vi "testCreate.vi"(8 "error in (no error)":errorcluster, 11 "TestCase in":refnum<class "StringList_Delegations.lvclass">) -> (0 "error out":errorcluster, 3 "TestCase out":refnum<class "StringList_Delegations.lvclass">)   [LabVIEW 2013, in "StringList_Delegations.lvclass"]
uses:
  StringList_Delegations.lvclass
  StringList_Delegations.lvclass/StringList_Delegations.ctl
  <vilib>/addons/_JKI Toolkits/VI Tester/TestCase.llb/TestCase.lvclass
  UnitTestComparisons/UnitTestComparisons.lvlib
  Test Doubles/ListImp_RefSpy/ListImp_RefSpy.lvclass
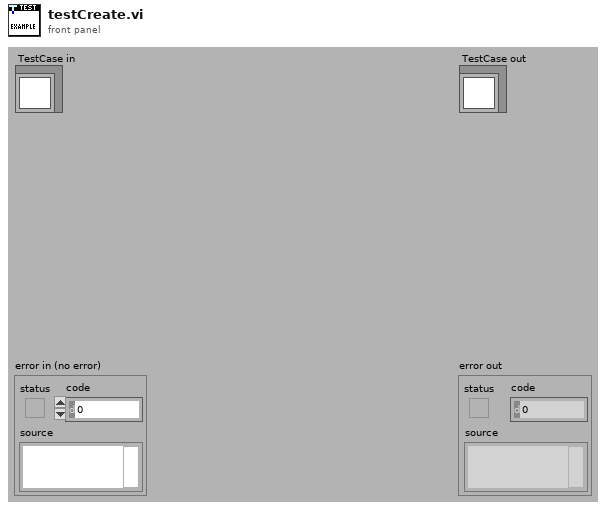
[diagram p1: front panel]
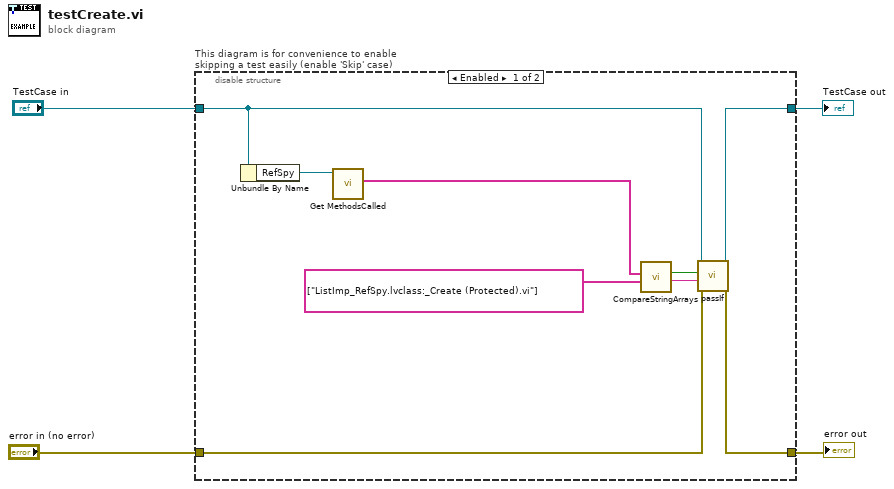
[diagram p0: block diagram]
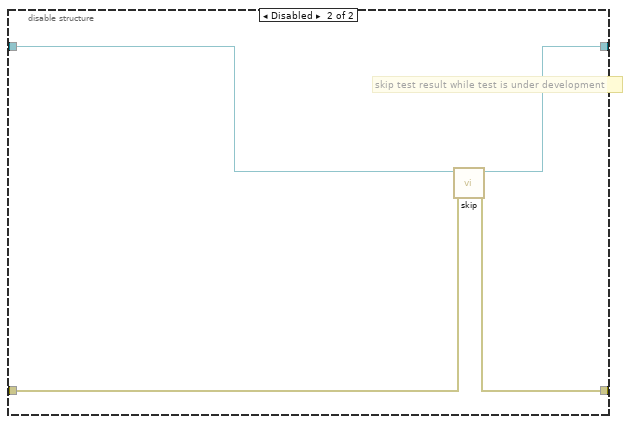
[diagram p2: hidden frame]
diagram:
  n1 = disable-structure "This diagram is for convenience to enable skipping a test easily (enable 'Skip' case)" shown="Enabled" {
    disable-tunnel: "TestCase in" -> [w7 w17]
    disable-tunnel: [w13 w15] -> w1
    disable-tunnel: [w12 w16] -> w3
    disable-tunnel: "error in (no error)" -> [w11 w14]
    frame Enabled {
      n2 = Unbundle By Name(w7) -> ("RefSpy"=w6:refnum<class "ListImp_RefSpy.lvclass">)
      n3 = call "Get MethodsCalled.vi"("MockListImp"=w6) -> ("MethodsCalled"=w5:string[])  [unwired: 9 in, 1 out]
      n4 = call "CompareStringArrays.vi"("Expected Strings"=string[] ["ListImp_RefSpy.lvclass:_Create (Protected).vi"] ("Actual Strings"), "Actual Strings"=w5) -> ("Message"=w9:string, "Equal?"=w10:bool)  [unwired: 8 in]
      n5 = call-dynamic "passIf.vi"("error in (no error)"=w11, "message (\"\")"=w9, "pass"=w10, "TestCase in"=w7) -> ("error out"=w12:errorcluster, "TestCase out"=w13:refnum<class "StringList_Delegations.lvclass">)  [unwired: 6 in]
    }
    frame Disabled {
      # "skip test result while test is under development"
      n6 = call <vilib>:"skip.vi"("error in (no error)"=w14, "TestCase in"=w17) -> ("error out"=w16:errorcluster, "TestCase out"=w15:refnum<class "StringList_Delegations.lvclass">)  [unwired: 8 in]
    }
  }
  "error out" <- w3
  "TestCase out" <- w1
